vi "Index_Array_2D.vi"(9 "Indexs IA":T1, 10 "Index Array 2D":i8[][](array[numeric])=[[0, 4, -3], [1, 5, -4], [2, -1, -5], [3, -2, 100]], 11 "E or S Index Array 2D":T2) -> (2 "Index SubArray":i8[](array[numeric]), 3 "Index Value":i8)   [LabVIEW 2018]
uses:
  Controls/E_S.ctl
  Controls/Rows_Columns.ctl
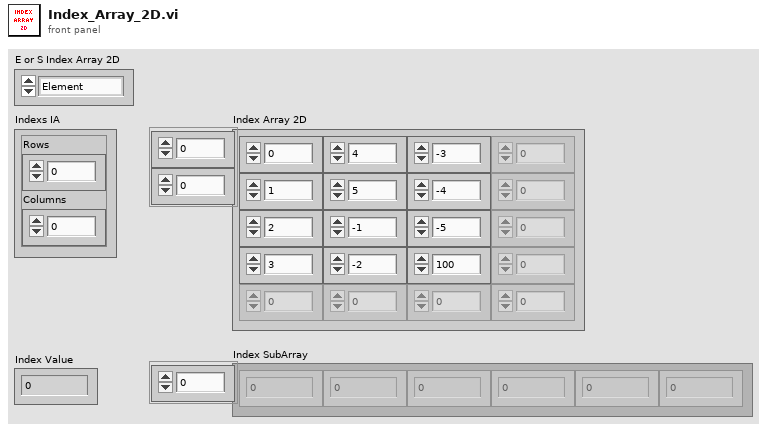
[diagram p1: front panel]
types:
  T1 = typedef "Rows_Columns.ctl" = cluster{"Rows":i32, "Columns":i32}
  T2 = typedef "E_S.ctl" = enum16{"Element", "SubArray"}
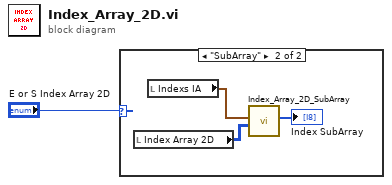
[diagram p0: block diagram]
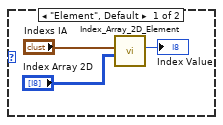
[diagram p2: hidden frame]
diagram:
  n1 = case shown="\"SubArray\"" "E or S Index Array 2D" {
    frame "Element", Default {
      n2 = call "Index_Array_2D_Element.vi"("Index Array 2D"="Index Array 2D", "Indexs IA"="Indexs IA") -> ("Value"=→"Index Value":i8)  [unwired: 9 in]
    }
    frame "SubArray" {
      n3 = local read "Index Array 2D"() -> (w5:i8[][])
      n4 = local read "Indexs IA"() -> (w6:T1)
      n5 = call "Index_Array_2D_SubArray.vi"("Index Array 2D"=w5, "Indexs IA"=w6) -> ("Index SubArray"=→"Index SubArray":i8[])  [unwired: 9 in]
    }
  }
